vi "Get Plugins from Configuration.vi"(8 "error in (no error)":errorcluster, 11 "Application Data In":T2) -> (0 "error out":errorcluster, 1 "Settings":T1[](array[typedef]), 2 "Items":T1[](array[typedef]), 3 "Application Data out":T2)   [LabVIEW 2017, in "DSF Configuration Utility.lvlib"]
uses:
  DSF Configuration Utility.lvlib
  Main VI/Application Data.ctl
  DSF/Data Sharing Framework Core/Data Sharing Framework Core.lvlibp/Configuration/1.0.0/Public/Controls/DSF Config Data RefNum.ctl
  Main VI/View Mode.ctl
  Tree Item.ctl
  Create New Tree Item.vi
  DSF/Data Sharing Framework Core/Data Sharing Framework Core.lvlibp/Configuration/1.0.0/Public/Read Item.vi
  DSF/Data Sharing Framework Core/Data Sharing Framework Core.lvlibp/Configuration/1.0.0/Public/Read Item/Read Settings.vi
  DSF/Data Sharing Framework Core/Data Sharing Framework Core.lvlibp/Configuration/1.0.0/Public/Read Item/Read Plugin.vi
  DSF/Data Sharing Framework Core/Data Sharing Framework Core.lvlibp/Configuration/1.0.0/Data Sharing Framework Configuration.lvlib
panel:
  # "App\nData"
  # "App\nData"
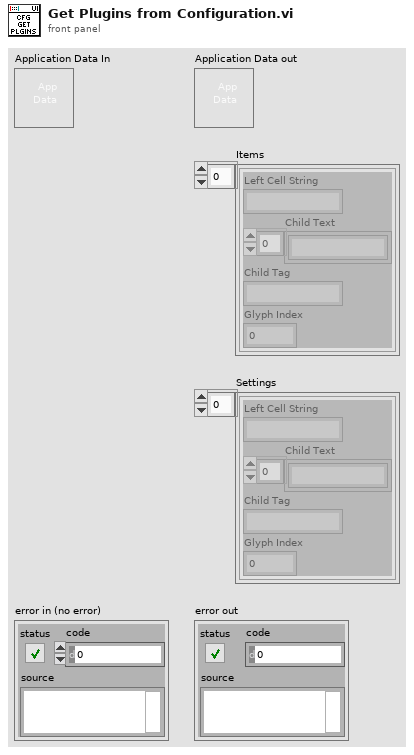
[diagram p1: front panel]
types:
  T1 = typedef "DSF Configuration Utility.lvlib/Tree Item.ctl" = cluster{"Left Cell String":string, "Child Text":string[], "Child Tag":string, "Glyph Index":i32}
  T2 = typedef "DSF Configuration Utility.lvlib/Application Data.ctl" = cluster{"Item Tree Control":refnum<vi>, "Value Tree Control":refnum<vi>, "DSF Refnum":T3, "Top-Level VI":refnum<vi>, "View State":T4, "menu reference":refnum<k9>}
  T3 = typedef "Data Sharing Framework Core.lvlibp/Data Sharing Framework Configuration.lvlib/DSF Config Data RefNum.ctl" = refnum<k1>
  T4 = typedef "DSF Configuration Utility.lvlib/View Mode.ctl" = enum16{"Tree", "List"}
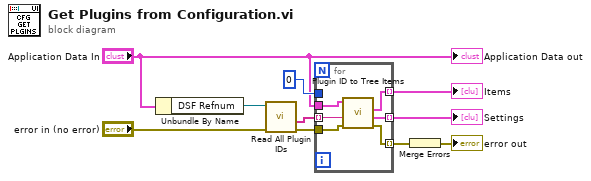
[diagram p0: block diagram]
diagram:
  n1 = Unbundle By Name("Application Data In") -> ("DSF Refnum"=w4:T3)
  n2 = call "Read All Plugin IDs.vi"("error in (no error)"="error in (no error)", "dsf refnum"=w4) -> ("error out"=w7:errorcluster, "Plugin IDs"=w8:string[])  [unwired: 7 in, 1 out]
  n3 = for {
    tunnel: w7 -> [w16]
    tunnel: w8 -> [w14] mode=indexing
    tunnel: [w15] -> w9 mode=indexing
    tunnel: 0 -> [_]
    tunnel: [w13] -> w2 mode=indexing
    tunnel: "Application Data In" -> [w12]
    tunnel: [w11] -> w1 mode=indexing
    n4 = call "Plugin ID to Tree Items.vi"("error in (no error)"=w16, "Plugin ID"=w14, "Application Data in"=w12) -> ("error out"=w15:errorcluster, "Settings"=w11:T1, "Item"=w13:T1)  [unwired: 5 in, 1 out]
  }
  "Items" <- w2
  "Settings" <- w1
  n5 = Merge Errors(w9) -> (→"error out":errorcluster)
  "Application Data out" <- "Application Data In"
